vi "AI端口_油压1.vi"() -> ()   [LabVIEW 2013]
panel:
  out "油压1":tag="Dev1/ai1"
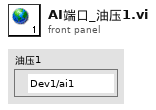
[diagram p1: front panel]
diagram:
